vi "Create 256 Values Palette.vi"(5 "Image High Color":u32(colorbox), 7 "Image Low Color":u32(colorbox), 9 "Source Image Display Range":cluster{"Min Value":dbl, "Max Value":dbl}={"Min Value"=nan, "Max Value"=nan}, 10 "Interpolate?":bool, 11 "Palette Colors in":u32[](array[colorbox])) -> (0 "Color Scale Marker Values":cluster{"Value":dbl, "Color":u32}[](array[cluster]), 2 "1D U32 array":u32[](array[colorbox]), 3 "1D Color value array":cluster{"Red":u8, "Green":u8, "Blue":u8}[](array[cluster]))   [LabVIEW 2021]
uses:
  <vilib>/vision/NI_Vision_Development_Module.lvlib
panel:
  out "Color Ramp":dbl(ramp)
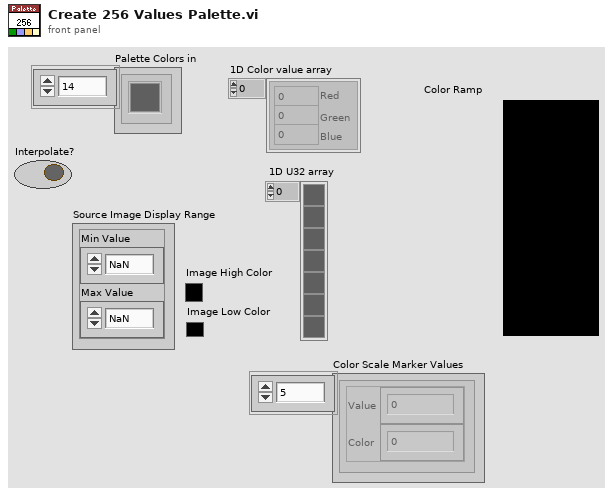
[diagram p1: front panel]
types:
  T1 = typedef "For Loop Iteration Type.ctl" = enum16{"default", "first", "last", "out of range"}
  T2 = cluster{"Red (or Hue) value":u8, "Green (or Sat) value":u8, "Blue (or Light or Val) value":u8}[]
  T3 = cluster{"Red (or Hue) value":u8, "Green (or Sat) value":u8, "Blue (or Light or Val) value":u8}
  T4 = cluster{"Numeric Control":dbl, "Numeric Control":u32}
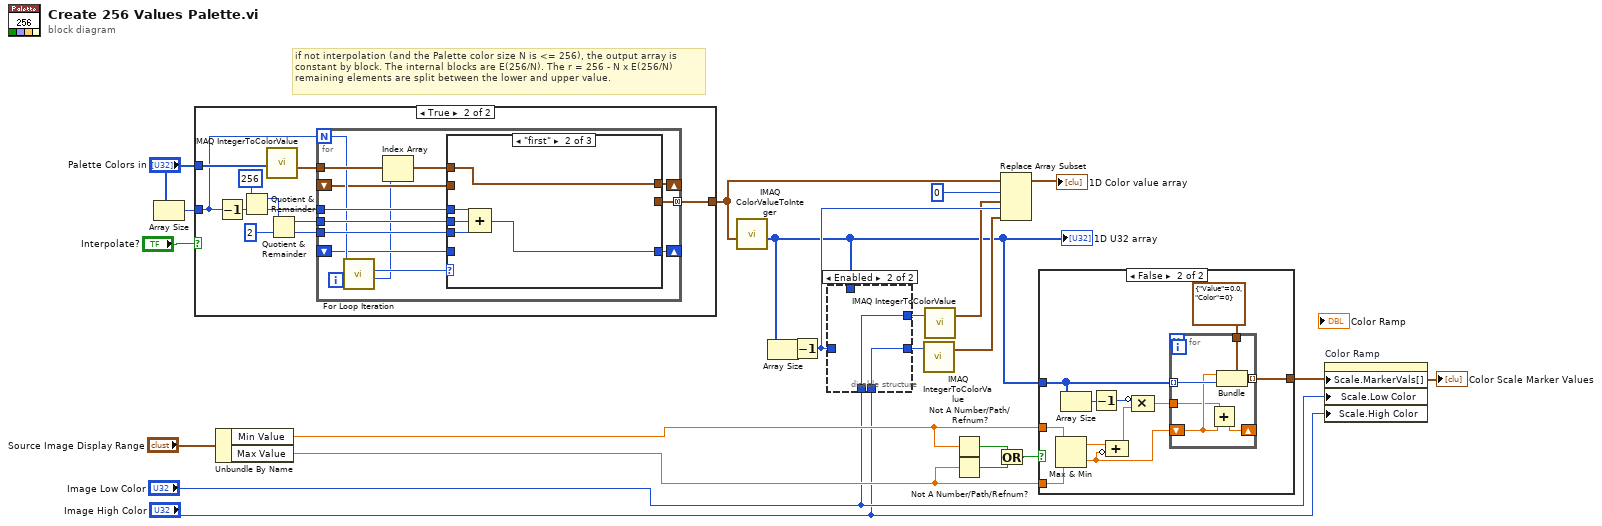
[diagram p0: block diagram]
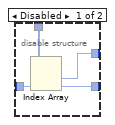
[diagram p2: hidden frame]
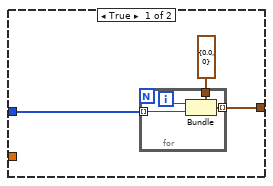
[diagram p3: hidden frame]
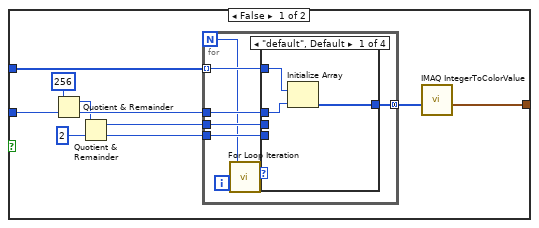
[diagram p4: hidden frame]
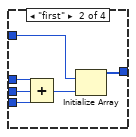
[diagram p5: hidden frame]
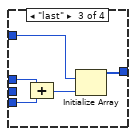
[diagram p6: hidden frame]
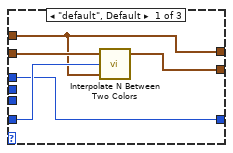
[diagram p8: hidden frame]
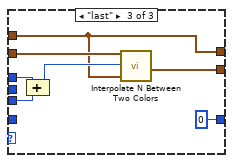
[diagram p9: hidden frame]
diagram:
  # "if not interpolation (and the Palette color size N is <= 256), the output array is\nconstant by block. The internal blocks are E(256/N). The r = 256 - N x E(256/N)\nremaining elements are split between the lower and upper value."
  n1 = Array Size(array="Palette Colors in") -> (size(s)=w21:i32)
  n2 = case shown="True" "Interpolate?" {
    tunnel: w21 -> [w32 w56]
    tunnel: "Palette Colors in" -> [w27 w59]
    tunnel: [w23 w57] -> w11
    frame False {
      n3 = Quotient & Remainder(x=256, y=w32) -> (x-y*floor(x/y)=w30:i32, floor(x/y)=w31:i32)
      n4 = Quotient & Remainder(x=w30, y=2) -> (x-y*floor(x/y)=w28:i32, floor(x/y)=w26:i32)
      n5 = for {
        N -> [w33]
        tunnel: w31 -> [w38]
        tunnel: w26 -> [w40]
        tunnel: w28 -> [w39]
        tunnel: w27 -> [w36] mode=indexing
        tunnel: [w37] -> w24 mode=concatenating
        i -> [w35]
        n6 = call "For Loop Iteration.vi"("i"=w35, "N"=w33) -> ("Iteration"=w34:T1)  [unwired: 8 in, 1 out]
        n7 = case shown="\"default\", Default" w34 {
          tunnel: w40 -> [_ w49 w54 _]
          tunnel: w39 -> [_ w48 _ _]
          tunnel: w38 -> [w43 w47 w53 _]
          tunnel: w36 -> [w42 w45 w51 _]
          tunnel: [w41 w44 w50 _] -> w37
          frame "default", Default {
            n8 = Initialize Array(w42, w43) -> (w41:u32[])
          }
          frame "first" {
            n9 = Compound Arithmetic op=ADD(w47, w48, w49) -> (w46:i32)
            n10 = Initialize Array(w45, w46) -> (w44:u32[])
          }
          frame "last" {
            n11 = Compound Arithmetic op=ADD(w53, w54) -> (w52:i32)
            n12 = Initialize Array(w51, w52) -> (w50:u32[])
          }
          frame "out of range" {
          }
        }
      }
      n13 = call "IMAQ IntegerToColorValue"("1D U32 array"=w24) -> ("1D Color value array"=w23:T2)  [unwired: 4 in, 3 out]
    }
    frame True {
      n14 = Decrement(x=w56) -> (x-1=w55:i32)
      n15 = Quotient & Remainder(x=256, y=w55) -> (x-y*floor(x/y)=w64:i32, floor(x/y)=w65:i32)
      n16 = call "IMAQ IntegerToColorValue"("1D U32 array"=w59) -> ("1D Color value array"=w58:T2)  [unwired: 4 in, 3 out]
      n17 = Quotient & Remainder(x=w64, y=2) -> (x-y*floor(x/y)=w62:i32, floor(x/y)=w61:i32)
      n18 = for {
        N: w56 -> [w75]
        tunnel: w65 -> [w77]
        tunnel: w61 -> [w79]
        tunnel: w62 -> [w78]
        tunnel: w58 -> [w76]
        shift-right: [w72] -> _
        shift-left: _ -> [w70]
        shift-right: [w71] -> _
        shift-left: _ -> [w69]
        tunnel: [w68] -> w57 mode=concatenating
        i -> [w74]
        n19 = call "For Loop Iteration.vi"("i"=w74, "N"=w75) -> ("i (dup)"=w66:i32, "Iteration"=w73:T1)  [unwired: 8 in]
        n20 = Index Array(array=w76, index=w66) -> (element=w67:T3)
        n21 = case shown="\"first\"" w73 {
          tunnel: w79 -> [_ w89 w96]
          tunnel: w78 -> [_ w88 _]
          tunnel: w77 -> [w82 w87 w95]
          tunnel: w67 -> [w80 w86 w91]
          tunnel: [w80 w86 w91] -> w72
          tunnel: [w82 w85 0] -> w71
          tunnel: w70 -> [w81 _ w92]
          tunnel: w69 -> [w83 _ _]
          tunnel: [w84 _ w94] -> w68
          frame "default", Default {
            n22 = call "Interpolate N Between Two Colors.vi"("Starting Color Value"=w81, "# Elements"=w83, "Ending Color Value"=w80) -> ("Color Array"=w84:T2)  [unwired: 6 in]
          }
          frame "first" {
            n23 = Compound Arithmetic op=ADD(w87, w88, w89) -> (w85:i32)
          }
          frame "last" {
            n24 = Compound Arithmetic op=ADD(w95, w96) -> (w93:i32)
            n25 = call "Interpolate N Between Two Colors.vi"("Starting Color Value"=w92, "# Elements"=w93, "Ending Color Value"=w91) -> ("Color Array"=w94:T2)  [unwired: 6 in]
          }
        }
      }
    }
  }
  n26 = Unbundle By Name("Source Image Display Range") -> ("Min Value"=w16:dbl, "Max Value"=w15:dbl)
  n27 = call "IMAQ ColorValueToInteger"("1D Color value array"=w11) -> ("1D U32 array"=w3:u32[])  [unwired: 4 in, 3 out]
  "1D U32 array" <- w3
  n28 = Array Size(array=w3) -> (size(s)=w12:i32)
  n29 = Decrement(x=w12) -> (x-1=w9:i32)
  n30 = disable-structure shown="Enabled" {
    disable-tunnel: w9 -> [w100 _]
    disable-tunnel: [w99 w102] -> w5
    disable-tunnel: [w98 w101] -> w4
    disable-tunnel: w3 -> [w97 _]
    disable-tunnel: "Image Low Color" -> [_ w102]
    disable-tunnel: "Image High Color" -> [_ w101]
    frame Disabled {
      n31 = Index Array(array=w97, index #2=w100) -> (element #1=w99:u32, element #2=w98:u32)  [unwired: 1 in]
    }
    frame Enabled {
    }
  }
  n32 = call "IMAQ IntegerToColorValue"("U32 value"=w4) -> ("Color Value"=w7:T3)  [unwired: 4 in, 3 out]
  n33 = call "IMAQ IntegerToColorValue"("U32 value"=w5) -> ("Color Value"=w8:T3)  [unwired: 4 in, 3 out]
  n34 = Not A Number/Path/Refnum?(number/path/refnum=w16) -> (NaN/Path/Refnum?=w19:bool)
  n35 = Not A Number/Path/Refnum?(number/path/refnum=w15) -> (NaN/Path/Refnum?=w18:bool)
  n36 = Or(x=w19, y=w18) -> (x .or. y?=w13:bool)
  n37 = Replace Array Subset(array=w11, new element #1=w8, index #1=0 ("index"), new element #2=w7, index #2=w9) -> (→"1D Color value array":T2)
  n38 = case shown="False" w13 {
    tunnel: w3 -> [w105 w116]
    tunnel: [w104 w120] -> w14
    tunnel: w15 -> [_ w117]
    tunnel: w16 -> [_ w118]
    frame True {
      n39 = for {
        tunnel: w105 -> [w108] mode=indexing
        tunnel: [w107] -> w104 mode=indexing
        tunnel: T4 {"Numeric Control"=0.0, "Numeric Control"=0} ("Scale.Marker Values[]") -> [w106]
        i -> [w109]
        n40 = Bundle(cluster=w106, "Numeric Control"=w109, "Numeric Control"=w108) -> (w107:T4)
      }
    }
    frame False {
      n41 = Max & Min(x=w118, y=w117) -> (max(x,y)=w115:dbl, min(x,y)=w114:dbl)
      n42 = Array Size(array=w116) -> (size(s)=w111:i32)
      n43 = Decrement(x=w111) -> (x-1=w110:i32)
      n44 = Compound Arithmetic op=ADD(w115, invert w114) -> (w113:dbl)
      n45 = Compound Arithmetic op=MULTIPLY(invert w110, w113) -> (w112:dbl)
      n46 = for {
        tunnel: w116 -> [w126] mode=indexing
        tunnel: [w125] -> w120 mode=indexing
        tunnel: cluster{"Value":dbl, "Color":u32} {"Value"=0.0, "Color"=0} ("Scale.Marker Values[]") -> [w124]
        shift-right: [w121] -> _
        shift-left: w114 -> [w123]
        tunnel: w112 -> [w122]
        n47 = Add(x=w122, y=w123) -> (x+y=w121:dbl)
        n48 = Bundle(cluster=w124, "Value"=w123, "Color"=w126) -> (w125:cluster{"Value":dbl, "Color":u32})
      }
    }
  }
  "Color Scale Marker Values" <- w14
  n49 = property on="Color Ramp" class="ColRmp (strict)"("Scale.MarkerVals[]"=w14, "Scale.Low Color"="Image Low Color", "Scale.High Color"="Image High Color") -> ()  [unwired: 2 in, 2 out]
